vi "cam-draw-target-oval.vi"(11 "Refnum in":T1) -> (3 "Refnum out":T1)   [LabVIEW 2020]
uses:
  <vilib>/vision/Image Controls.llb/IMAQ Image.ctl
  <vilib>/Rock Robotics/Network Tables/NT Read Number.vi
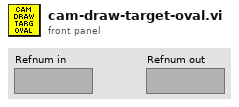
[diagram p1: front panel]
types:
  T1 = typedef "IMAQ Image.ctl" = refnum<image>
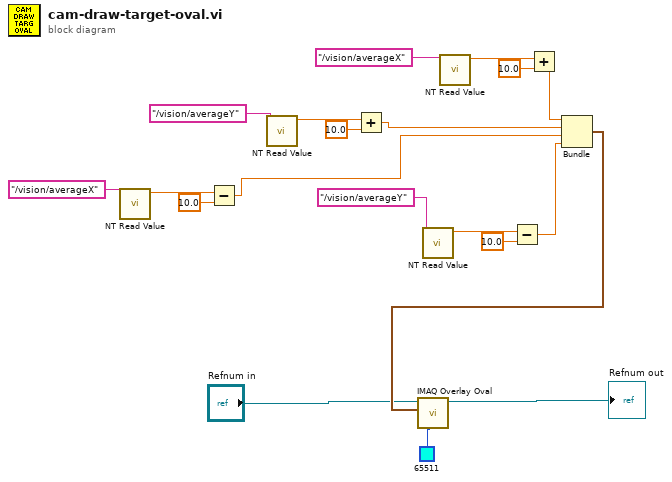
[diagram p0: block diagram]
diagram:
  n1 = call-poly <vilib>:"NT Read Value.vi"("name"="/vision/averageX" ("Name")) -> ("value"=w8:dbl)  [unwired: 8 in, 2 out]
  n2 = Subtract(x=w8, y=10.0) -> (x-y=w18:dbl)
  n3 = call-poly <vilib>:"NT Read Value.vi"("name"="/vision/averageY" ("Name")) -> ("value"=w5:dbl)  [unwired: 8 in, 2 out]
  n4 = Add(x=w5, y=10.0) -> (x+y=w17:dbl)
  n5 = call-poly <vilib>:"NT Read Value.vi"("name"="/vision/averageY" ("Name")) -> ("value"=w14:dbl)  [unwired: 8 in, 2 out]
  n6 = call-poly <vilib>:"NT Read Value.vi"("name"="/vision/averageX" ("Name")) -> ("value"=w11:dbl)  [unwired: 8 in, 2 out]
  n7 = Subtract(x=w14, y=10.0) -> (x-y=w19:dbl)
  n8 = Add(x=w11, y=10.0) -> (x+y=w16:dbl)
  n9 = Bundle(w16, w17, w18, w19) -> (w20:cluster{dbl, dbl, dbl, dbl})  [unwired: 1 in]
  n10 = call "IMAQ Overlay Oval"("Color"=u32 65511, "Bounding Rectangle"=w20, "Image"="Refnum in") -> ("Image Out"=→"Refnum out":T1)  [unwired: 7 in, 1 out]
